vi "CheckCHconfig.vi"(0 "Trigger":T3(ring), 5 "Source":T1=-2147483648 items=["[read only]"=-2147483648, "ADC 1"=0, "ADC 2"=1, "ADC 3"=2, "ADC 4"=3, "ADC 5"=4, "ADC 6"=5, "HF 1 Out"=7, "HF 1 df"=8, "z out"=9, "HF 1"=12, "HF 1 Ampl."=13, "HF 1 Phase"=14, "LF LockIn Ampl"=16, "LF LockIn Phase"=17, "z out inv"=18, "counter"=23, "Crosslink 1"=29, "Crosslink 2"=30, "Pos X"=31, "Pos Y"=32], 11 "error in":T2) -> (4 "Corresponding channels":i32[](array[numeric]), 6 "Corresponding trig_sources":i32[](array[numeric]), 8 "Corresponding sources":i32[](array[numeric]), 15 "error out":T2)   [LabVIEW 2016]
doc: "This VI provides information about the configuration of the fourteen data channel regarding one of the input variables. Apart from the error in cluster it has two input variables. Trigger defines the event that causes data acquisition on a specific channel. \"Source\" defines where the data comes from. It works as follows. If you connect a specific trigger VI-input of the same name, the VI will output arrays with different content:\n-\"Corresponding channels\" contains the numbers of channel (0-13) that are triggered by the given input.\n-\"channels\" is an array filled with 14 numbers that are either -1 or 1. The index of the array element equals the channel number. If the element of index 4 equals 1, it means that channel 4 is triggered by the same trigger specified by the input-variable \"Trigger\". If the array element of index 4 equals -1 it means, that channel 4 is triggered by a different as the requested trigger.\n-\"Corresponding trig_sources\" contains the sources that are set to the requested trigger in any channel. The numbers in the array represent the sources as defined in the typedef \"channel-source_selection\".\n-\"trig_sources\" is an array of 14 elements which contains either a -1 or a number representing the source of the channel as defined in the typedef \"channel-source_selection\". The index of the array where the number is located tells you which channel is set to the configuration. If there is the number -1 at the array index 4, it means that channel 5 is set to a different trigger as the input \"Trigger\". If the array contains the number 3 at index 4, it means that channel 5 is set to the same trigger as the input \"Trigger\" and that channel five is set to the source \"ADC 4\" (see typedef \"channel-source_selection\").\nIf the input \"source\" is connected, the VI provides information about the channel configuration in the following arrays:\n-The array \"Corresponding sources\" contains the numbers of channels that are set to retrieve data from the \"source\" given by the input variable \"Source\".\n-\"sources\" is an array of 14 elements that works similar to \"channels\" with the difference that it checks the sources instead of triggers."
uses:
  Controls/Error_Out.ctl
  Controls/Channel-Source_Selection.ctl
  Files_ASC500/DLL/ASC500_RemoteControlV27.dll
panel:
  out "sources":i32[](array[numeric])
  out "trig_source":i32[](array[numeric])
  out "channels":i32[](array[numeric])
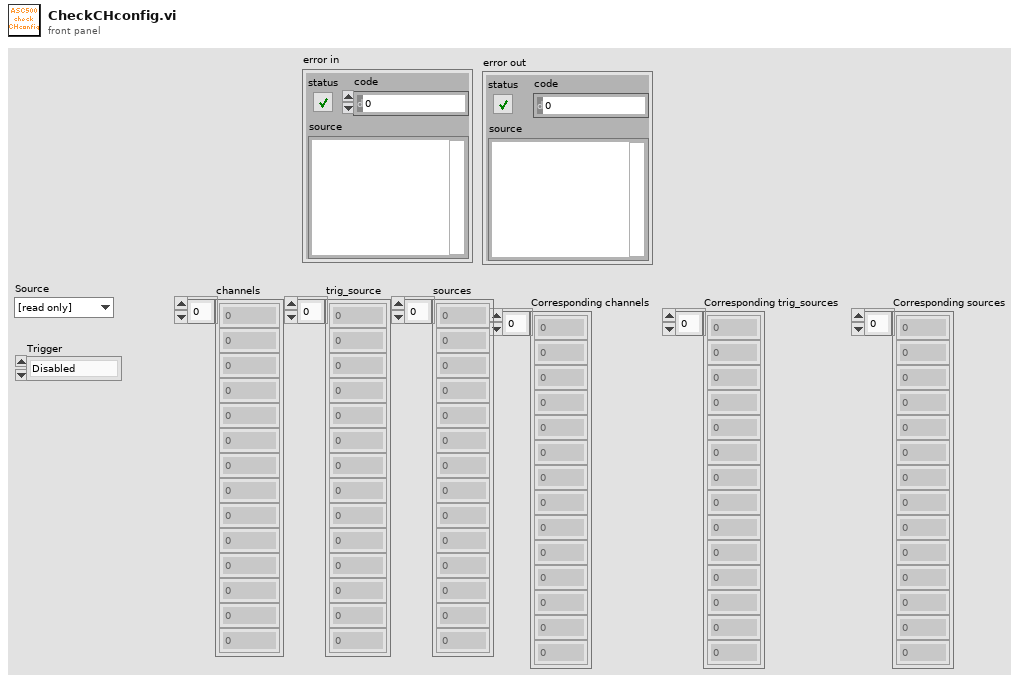
[diagram p1: front panel]
types:
  T1 = typedef "Channel-Source_Selection.ctl" = i32
  T2 = typedef "Error_Out.ctl" = errorcluster
  T3 = enum32{"Disabled", "Scan", "Line", "Spec 1", "Spec 2", "Spec 3", "Cal", "Trigger", "Every", "SoftSpec", "DualPass", "Step Scan"}
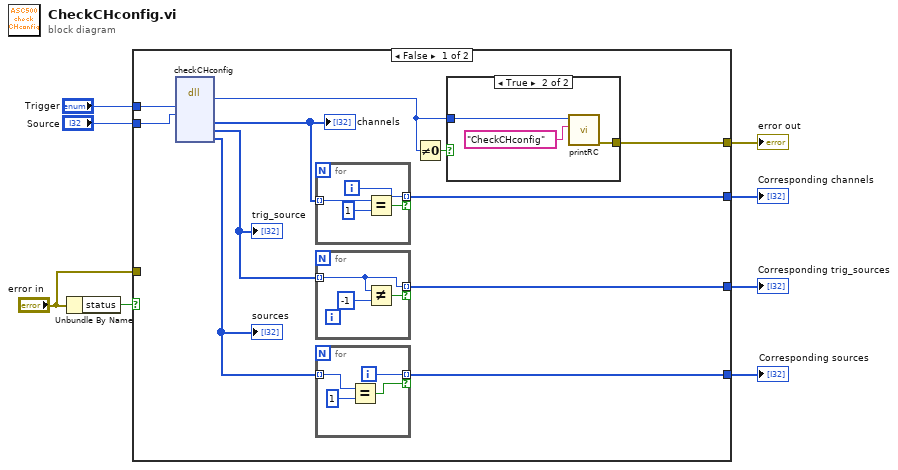
[diagram p0: block diagram]
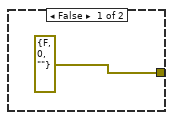
[diagram p2: hidden frame]
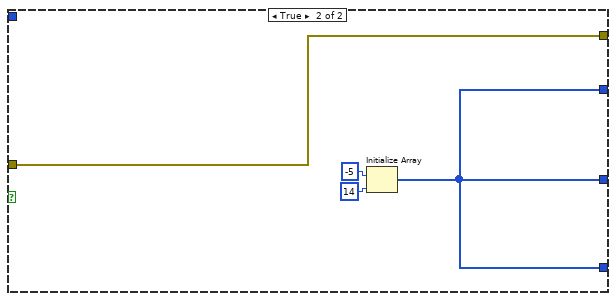
[diagram p3: hidden frame]
diagram:
  n1 = Unbundle By Name("error in") -> ("status"=w5:bool)
  n2 = case shown="False" w5 {
    tunnel: "error in" -> [_ w38]
    tunnel: [w18 w35] -> w8
    tunnel: [w15 w38] -> w7
    tunnel: "Trigger" -> [w14 _]
    tunnel: [w12 w35] -> w3
    tunnel: "Source" -> [w11 _]
    tunnel: [w9 w35] -> w2
    frame False {
      n3 = dll-call lib="G:/SCMOperations/Share/ELE/Produkt Information/ASC500/04 Remote Control/02 development versions/2018Nov06/Files_ASC500/DLL/ASC500_RemoteControlV27.dll" fn="checkCHconfig"("reqtrigger"=w14, "reqsource"=w11) -> ("return type"=w16:i32, "channel"=w19:i32[], "trig_sources"=w13:i32[], "sources"=w10:i32[])  [unwired: 8 in, 2 out]
      "channels" <- w19
      "trig_source" <- w13
      "sources" <- w10
      n4 = for {
        tunnel: w19 -> [w33] mode=indexing
        tunnel: [w32] -> w18 mode=indexing if=w31
        i -> [w32]
        n5 = Equal?(x=w33, y=1) -> (x = y?=w31:bool)
      }
      n6 = for {
        tunnel: w13 -> [w24] mode=indexing
        tunnel: [w24] -> w12 mode=indexing if=w25
        n7 = Not Equal?(x=w24, y=-1) -> (x != y?=w25:bool)
      }
      n8 = for {
        tunnel: w10 -> [w23] mode=indexing
        tunnel: [w20] -> w9 mode=indexing if=w21
        i -> [w20]
        n9 = Equal?(x=w23, y=1) -> (x = y?=w21:bool)
      }
      n10 = Not Equal To 0?(x=w16) -> (x != 0?=w17:bool)
      n11 = case shown="True" w17 {
        tunnel: [errorcluster {FALSE, 0, ""} w30] -> w15
        tunnel: w16 -> [_ w29]
        frame False {
        }
        frame True {
          n12 = call "printRC.vi"("additional information"="CheckCHconfig", "RC"=w29) -> ("error out"=w30:T2)  [unwired: 9 in]
        }
      }
    }
    frame True {
      n13 = Initialize Array(-5 ("element"), 14 ("dimension size")) -> (w35:i32[])
    }
  }
  "Corresponding channels" <- w8
  "error out" <- w7
  "Corresponding trig_sources" <- w3
  "Corresponding sources" <- w2
